vi "DSF.Transceiver.GE Reflective Memory.Set Transfer Group Parameters.vi"(10 "Transfer Group Parameters":T1[](array[typedef]), 11 "GE Reflective Memory in":refnum<class "DSF.Transceiver.GE Reflective Memory.lvclass">) -> (3 "GE Reflective Memory out":refnum<class "DSF.Transceiver.GE Reflective Memory.lvclass">)   [LabVIEW 2017, in "DSF.Transceiver.GE Reflective Memory.lvlib" / "DSF.Transceiver.GE Reflective Memory.lvclass"]
uses:
  DSF.Transceiver.GE Reflective Memory.lvclass
  DSF.Transceiver.GE Reflective Memory.Transfer Group Parameters.ctl
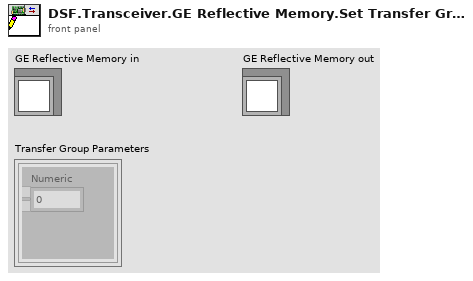
[diagram p1: front panel]
types:
  T1 = typedef "DSF.Transceiver.GE Reflective Memory.lvlib/DSF.Transceiver.GE Reflective Memory.lvclass/DSF.Transceiver.GE Reflective Memory.Transfer Group Parameters.ctl" = cluster{"Numeric":dbl}
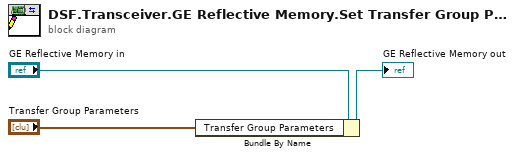
[diagram p0: block diagram]
diagram:
  n1 = Bundle By Name(cluster="GE Reflective Memory in", "Transfer Group Parameters"="Transfer Group Parameters") -> (→"GE Reflective Memory out":refnum<class "DSF.Transceiver.GE Reflective Memory.lvclass">)
